vi "XIPIN_Video_Scaler_3_0.vi"   [LabVIEW 2017]
doc: "The Xilinx Video Scaler LogicCORE is a sophisticated module that can spatially up-scale or down-scale video streams in real time. It can be configured to support conversions across all SD and HD resolutions from QCIF to 1080P and beyond. The core is implemented as a polyphase filter that supports 2-12 horizontal and vertical taps with programmable coefficients. The user may select either a parameterizable EDK PCore, a General Purpose Processor (GPP) interface netlist or a Constant interface netlist. The GPP and PCore interfaces enable a microprocessor to load coefficient sets in real time and program other scaler parameters.\n------------------------------------\n<b>Need License</b> : Yes"
uses:
  <vilib>/rvi/XilinxIP/XIPIN_XNode/niFpgaXIPIN.xnode
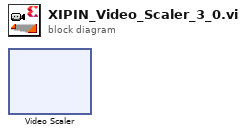
[diagram p0: block diagram]
diagram:
  n1 = xnode ("Video Scaler")() -> ()
